vi "Check_Position_PN.vi"(0 "Traverse Name":string, 1 "Collision mode":T1=enum."Traverse - All", 2 "Collision_detection":path=path "Please Run EnFlo Hub.vi", 5 "Position to check":sgl[](array[numeric])=[0.0, 0.0, 0.0] format="%.2g", 7 "Traverse Active Parts":cluster{"X":bool, "XY":bool, "XYZ":bool}, 9 "Traverse extruded position":sgl[](array[numeric])=[0.0, 0.0, 0.0] format="%.2g", 11 "Model Rotation (deg)":sgl[](array[numeric])=[0.0, 0.0, 0.0] format="%.2g", 12 "Extrusion mode":bool, 14 "Get minimum separation within look-out sphere":bool, 15 "Visualisation only (no collision detection)":bool) -> (3 "Collision":bool, 4 "Error Comments":string, 6 "Minimum separation":sgl, 8 "Traverse collision part":cluster{"X":bool, "XY":bool, "XYZ":bool}, 10 "Minimum separation vector (from trav.)":sgl[](array[numeric]))   [LabVIEW 2018]
uses:
  Collision_Detection/Triangles/EnFlo specific/Collision Mode.ctl
  <vilib>/Analysis/coordinate.llb/Euler Rotation Order.ctl
  <vilib>/Analysis/coordinate.llb/3D Cartesian Coordinate Rotation (Euler) (Scalar).vi
  <vilib>/Analysis/baseanly.llb/Unit Vector (DBL).vi
  <vilib>/Analysis/baseanly.llb/Real Dot Product.vi
  Collision_Detection/Triangles/EnFlo specific/Collision Detection global.vi
  <vilib>/Analysis/NI_AALPro.lvlib
  <vilib>/Analysis/NI_AALBase.lvlib
panel:
  out "Error out":errorcluster
  in  "3D graphics output":bool=TRUE
  # "X\n\nY\n\nZ"
  # "Roll\n\nPitch\n\nYaw"
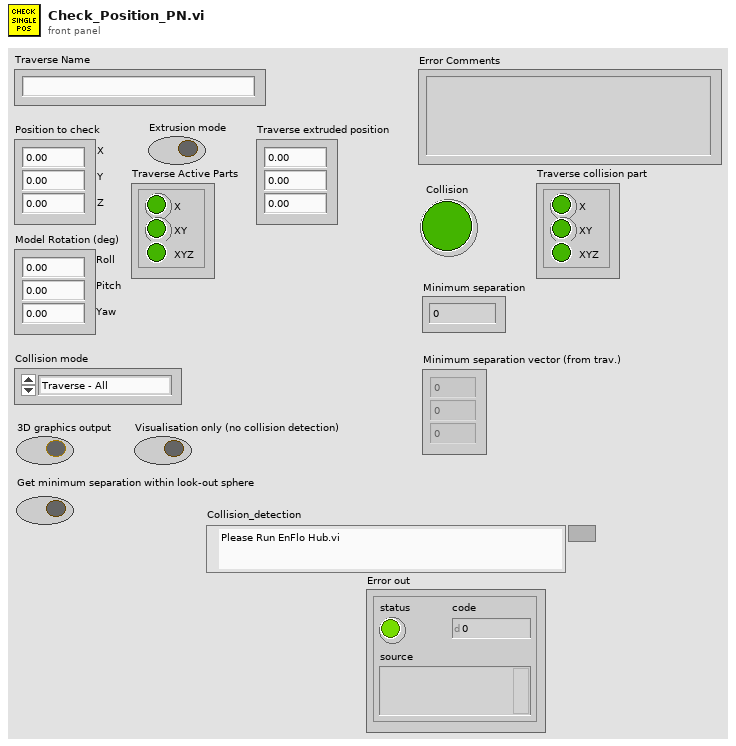
[diagram p1: front panel]
types:
  T1 = typedef "Collision Mode.ctl" = enum16{"Traverse - Tunnel", "Traverse - Model", "Traverse - Fixed objects", "Traverse - Traverse", "Traverse - All"}
  T2 = cluster{"Traverse Name":string, "Position to check":sgl[], "Model Rotation (deg)":sgl[], "Collision_detection":path, "Collision mode":T1, "Get minimum separation within look-out sphere":bool, "3D graphics output":bool, "Visualisation only (no collision detection)":bool, "Extrusion mode":bool, "Traverse extruded position":sgl[]}
  T3 = typedef "NI_AALPro.lvlib/Euler Rotation Order.ctl" = u16
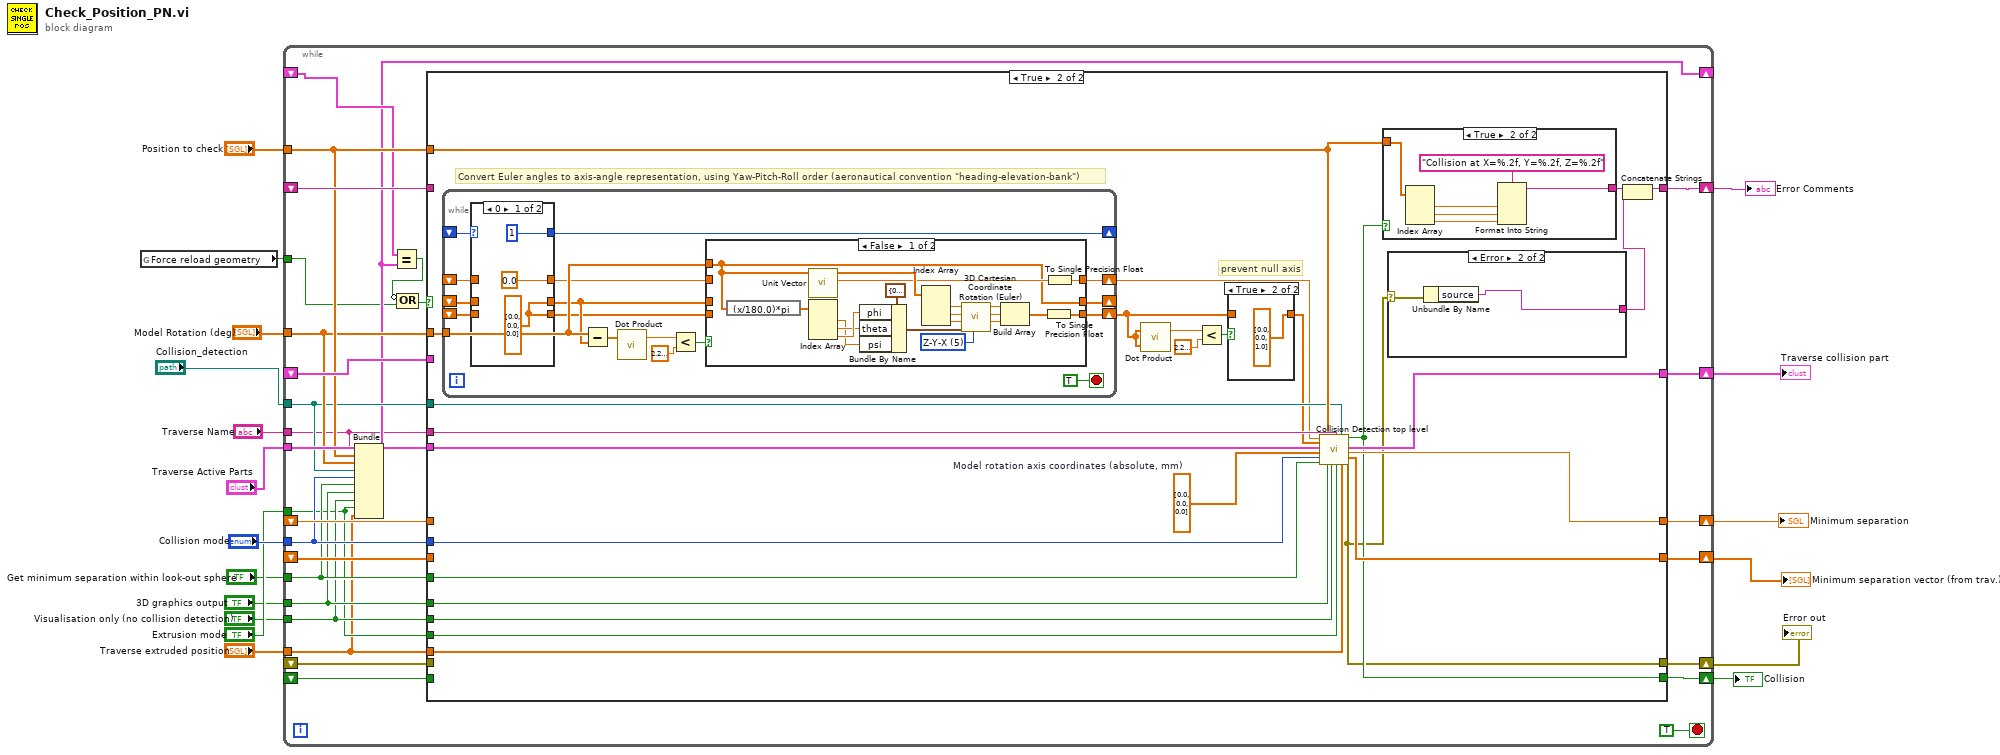
[diagram p0: block diagram]
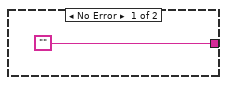
[diagram p3: hidden frame]
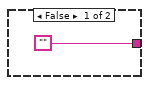
[diagram p7: hidden frame]
diagram:
  n1 = global read "Collision Detection global.vi" "Force reload geometry"() -> (w1:bool)
  n2 = while {
    tunnel: "Traverse Name" -> [w24]
    tunnel: "Position to check" -> [w36]
    tunnel: "Collision_detection" -> [w34]
    tunnel: "Collision mode" -> [w33]
    tunnel: "Extrusion mode" -> [w29]
    tunnel: "Traverse extruded position" -> [w28]
    tunnel: "3D graphics output" -> [w31]
    tunnel: "Visualisation only (no collision detection)" -> [w30]
    tunnel: "Model Rotation (deg)" -> [w35]
    shift-right: [w45] -> w4
    shift-left: _ -> [w41]
    shift-right: [w44] -> w5
    shift-left: _ -> [w40]
    shift-right: [w46] -> w8
    shift-left: _ -> [w39]
    shift-right: [w43] -> w6
    shift-left: _ -> [w38]
    shift-right: [w42] -> w7
    shift-left: _ -> [w37]
    tunnel: "Traverse Active Parts" -> [w47]
    tunnel: "Get minimum separation within look-out sphere" -> [w32]
    shift-right: [w26] -> _
    shift-left: _ -> [w27]
    shift-right: [w23] -> w2
    shift-left: _ -> [w22]
    tunnel: w1 -> [w19]
    stop <- TRUE stop-if-true
    n3 = Bundle("Traverse Name"=w24, "Position to check"=w36, "Model Rotation (deg)"=w35, "Collision_detection"=w34, "Collision mode"=w33, "Get minimum separation within look-out sphere"=w32, "3D graphics output"=w31, "Visualisation only (no collision detection)"=w30, "Extrusion mode"=w29, "Traverse extruded position"=w28) -> (w26:T2)  [unwired: 1 in]
    n4 = Equal?(x=w27, y=w26) -> (x = y?=w21:bool)
    n5 = Compound Arithmetic op=OR(invert w21, w19) -> (w20:bool)
    n6 = case shown="True" w20 {
      tunnel: w24 -> [_ w78]
      tunnel: w36 -> [_ w77]
      tunnel: [w53 w55] -> w45
      tunnel: w34 -> [_ w76]
      tunnel: w33 -> [_ w75]
      tunnel: w29 -> [_ w74]
      tunnel: w28 -> [_ w73]
      tunnel: w31 -> [_ w72]
      tunnel: w30 -> [_ w71]
      tunnel: w35 -> [_ w70]
      tunnel: [w50 w63] -> w43
      tunnel: [w49 w62] -> w42
      tunnel: [w52 w61] -> w44
      tunnel: w47 -> [_ w60]
      tunnel: w32 -> [_ w59]
      tunnel: [w51 w58] -> w46
      tunnel: w41 -> [w53 _]
      tunnel: w40 -> [w52 _]
      tunnel: w39 -> [w51 _]
      tunnel: w38 -> [w50 _]
      tunnel: w37 -> [w49 _]
      tunnel: [w48 w57] -> w23
      tunnel: w22 -> [w48 _]
      frame False {
      }
      frame True {
        w79 = sgl[] [0.0, 0.0, 0.0]  # Model rotation axis coordinates (absolute, mm)
        # "prevent null axis"
        # "Convert Euler angles to axis-angle representation, using Yaw-Pitch-Roll order (aeronautical convention \"heading-elevation-bank\")"
        n7 = while {
          shift-right: [w97] -> _
          shift-left: _ -> [w87]
          tunnel: w70 -> [w98]
          shift-right: [w100] -> w65
          shift-left: _ -> [w85]
          shift-right: [w96] -> w69
          shift-left: _ -> [w89]
          shift-right: [w91] -> _
          shift-left: _ -> [w92]
          stop <- TRUE stop-if-true
          n8 = case shown="0" w92 {
            selector: w92 -> [_ w108]
            tunnel: [u8 1 w108] -> w91
            tunnel: [sgl 0.0 w107] -> w90
            tunnel: w89 -> [_ w107]
            tunnel: [w102 w106] -> w88
            tunnel: w87 -> [_ w106]
            tunnel: [w102 w105] -> w86
            tunnel: w85 -> [_ w105]
            frame 0 {
              w102 = sgl[] [0.0, 0.0, 0.0]
            }
            frame Default {
            }
          }
          n9 = Subtract(x=w98, y=w88) -> (x-y=w94:sgl[])
          n10 = call-poly <vilib>:"Dot Product.vi"("X Vector"=w94) -> ("X * Y"=w93:dbl)  [unwired: 1 in, 1 out]
          n11 = Less?(x=w93, y=2.220446049250313e-16) -> (x < y?=w95:bool)
          n12 = case shown="False" w95 {
            tunnel: w98 -> [w111 _]
            tunnel: w88 -> [_ w130]
            tunnel: [w110 w129] -> w100
            tunnel: [w111 w130] -> w97
            tunnel: w86 -> [_ w129]
            tunnel: [w109 w128] -> w96
            tunnel: w90 -> [_ w128]
            frame False {
              w114 = T3 5 items=["X-Y-Z", "X-Z-Y", "Y-X-Z", "Y-Z-X", "Z-X-Y", "Z-Y-X", "X-Y-X", "X-Z-X", "Y-X-Y", "Y-Z-Y", "Z-X-Z", "Z-Y-Z"] ("rotation order")
              n13 = expression code="(x/180.0)*pi" ("degrees to radians")(w111) -> (w119:sgl[])
              n14 = call-poly <vilib>:"Unit Vector.vi"("Input Vector"=w111) -> ("norm"=w112:dbl, "Unit Vector"=w124:dbl[])  [unwired: 8 in, 1 out]
              n15 = Index Array(array=w119) -> (element #1=w120:sgl, element #2=w121:sgl, element #3=w122:sgl)  [unwired: 3 in]
              n16 = Bundle By Name(cluster=cluster{"phi":dbl, "theta":dbl, "psi":dbl} {"phi"=0.0, "theta"=0.0, "psi"=0.0} ("Euler Angles"), "phi"=w122, "theta"=w121, "psi"=w120) -> (w123:cluster{"phi":dbl, "theta":dbl, "psi":dbl})
              n17 = Index Array(array=w124) -> (element #1=w127:dbl, element #2=w126:dbl, element #3=w125:dbl)  [unwired: 3 in]
              n18 = call-poly <vilib>:"3D Cartesian Coordinate Rotation (Euler).vi"("rotation order"=w114, "Euler Angles"=w123, "z"=w125, "y"=w126, "x"=w127) -> ("z out"=w117:dbl, "y out"=w116:dbl, "x out"=w115:dbl)  [unwired: 3 in, 1 out]
              n19 = Build Array(w115, w116, w117) -> (w113:dbl[])
              n20 = To Single Precision Float(number=w113) -> (single precision float=w110:sgl[])
              n21 = To Single Precision Float(number=w112) -> (single precision float=w109:sgl)
            }
            frame True {
            }
          }
        }
        n22 = call-poly <vilib>:"Dot Product.vi"("Y Vector"=w65, "X Vector"=w65) -> ("X * Y"=w68:dbl)  [unwired: 1 out]
        n23 = Less?(x=w68, y=2.220446049250313e-16) -> (x < y?=w66:bool)
        n24 = case shown="True" w66 {
          tunnel: w65 -> [w83 _]
          tunnel: [w83 sgl[] [0.0, 0.0, 1.0]] -> w64
          frame False {
          }
          frame True {
          }
        }
        n25 = call "Collision Detection top level.vi"("Model rotation (degrees)"=w69, "Model rotation axis (unit vector)"=w64, "Traverse Active Parts"=w60, "Model rotation axis coordinates (absolute, mm)"=w79, "Collision mode"=w75, "Get minimum separation within look-out sphere"=w59, "Traverse position (absolute, mm)"=w77, "3D graphics output"=w72, "Visualisation only (no collision detection)"=w71, "Traverse name"=w78, "Extrusion mode"=w74, "Rig geometry directory path"=w76, "Traverse extruded position"=w73) -> ("Collision"=w58:bool, "Traverse collision part"=w61:cluster{"X":bool, "XY":bool, "XYZ":bool}, "Minimum separation"=w63:sgl, "Minimum separation vector (from trav.)"=w62:sgl[], "Error out"=w57:errorcluster)  [unwired: 1 in, 1 out]
        n26 = case shown="True" w58 {
          tunnel: w77 -> [_ w137]
          tunnel: ["" w132] -> w56
          frame False {
          }
          frame True {
            n27 = Index Array(array=w137) -> (element #1=w136:sgl, element #2=w135:sgl, element #3=w134:sgl)  [unwired: 3 in]
            n28 = Format Into String(format string="Collision at X=%.2f, Y=%.2f, Z=%.2f", w136, w135, w134) -> (resulting string=w132:string)  [unwired: 2 in, 1 out]
          }
        }
        n29 = case shown="Error" w57 {
          selector: w57 -> [_ w82]
          tunnel: ["" w81] -> w54
          frame No Error {
          }
          frame Error {
            n30 = Unbundle By Name(w82) -> ("source"=w81:string)
          }
        }
        n31 = Concatenate Strings(w56, w54) -> (w55:string)
      }
    }
  }
  "Collision" <- w8
  "Error Comments" <- w4
  "Minimum separation" <- w6
  "Minimum separation vector (from trav.)" <- w7
  "Traverse collision part" <- w5
  "Error out" <- w2
